vi "MotorControl_Test.vi"() -> ()   [LabVIEW 2020]
panel:
  out "Y Buffer":string
  in  "Y Axis Step Size":i32
  in  "Y Axis Range":i32
  out "Y Position":i32=2374 format="%b"
  out "Limit Switch Activated":bool
  out "Moving":bool
  out "Boolean Array":bool[](array[boolean])
  out "Binary Number":i32=2374 format="%b"
  in  "X Axis Step Size":i32
  in  "X Axis Range":i32
  in  "?":bool
  out "Angle Position":sgl
  out "X Position":sgl
  in  "Angle Step Size":i32
  in  "Angle Range":i32
  in  "?":refnum<k7>(container)
  out "X Translation Serial Number":i32=40849496
  in  "?":refnum<k7>(container)
  out "Angle Serial Number":i32=40808764
  # "Rotation Motor"
  # "Translation Motor"
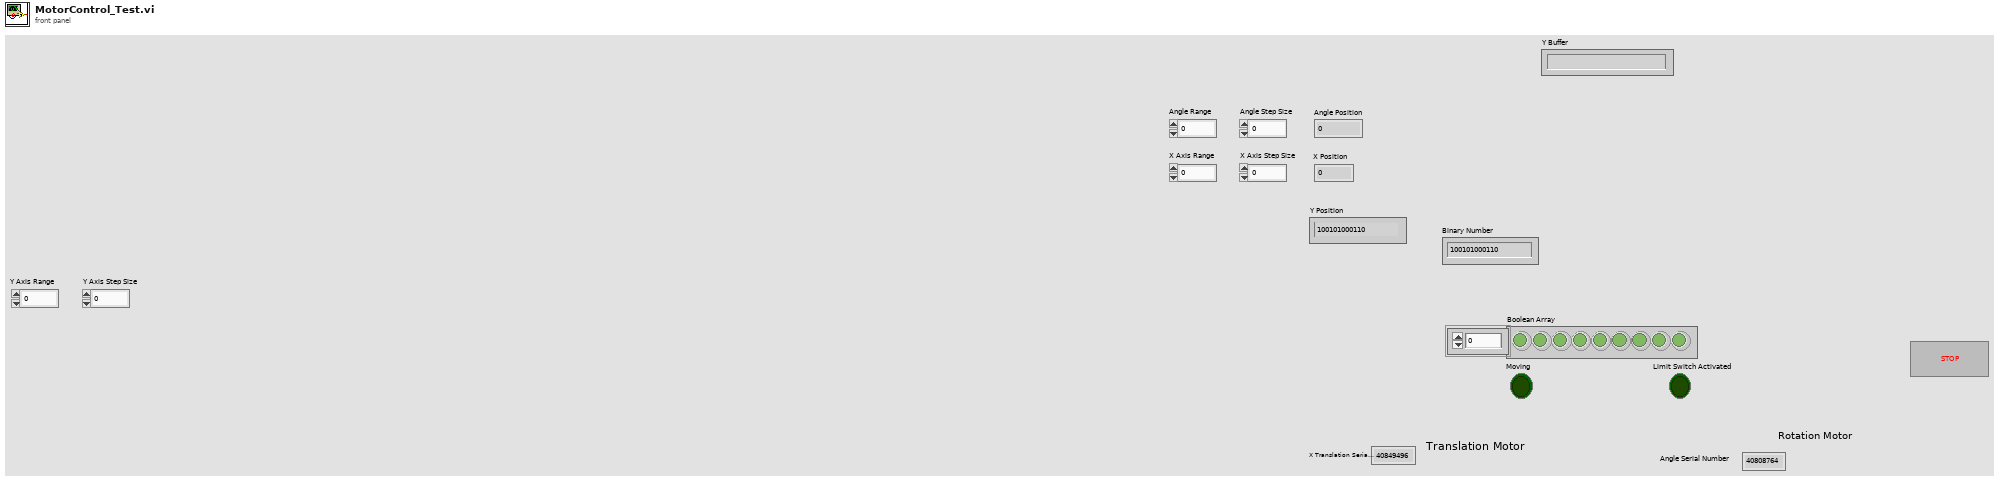
[diagram p1: front panel]
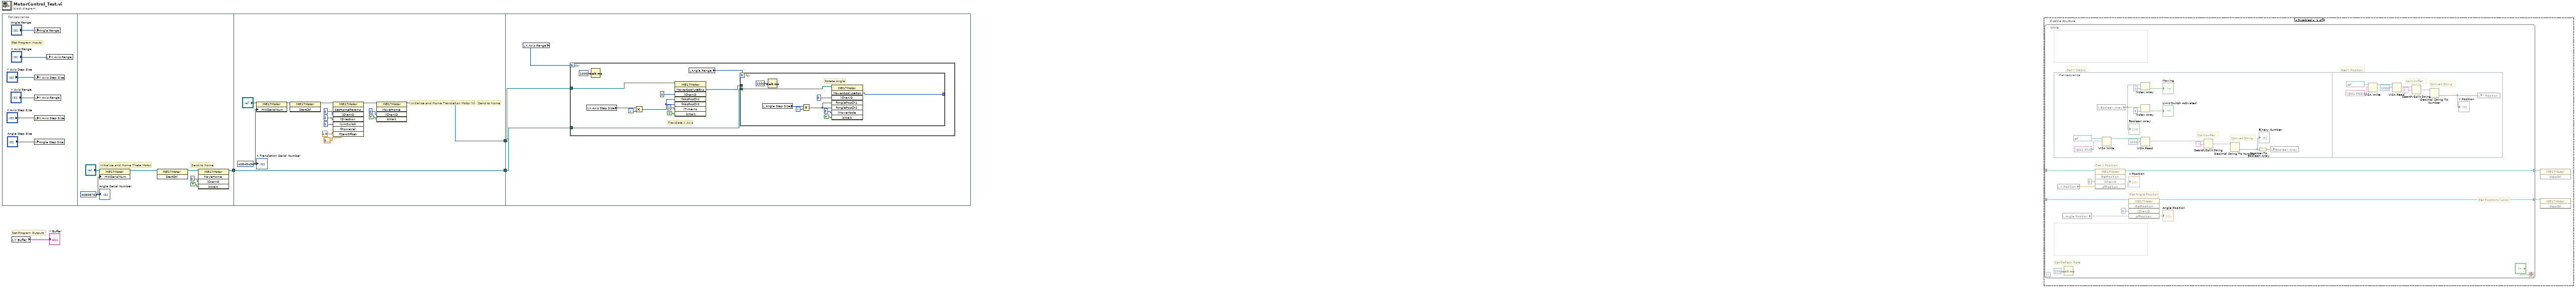
[diagram p0: block diagram]
diagram:
  # "Set Program Outputs"
  n1 = flat-sequence {
    tunnel: [w11] -> w4
    tunnel: w4 -> [w31]
    tunnel: [w31] -> w2
    tunnel: [w18] -> w1
    tunnel: w2 -> [w33]
    tunnel: w1 -> [w34]
    frame #0 {
      # "Get Program Inputs"
      n2 = local write "Angle Range"("Angle Range") -> ()
      n3 = local write "Y Axis Step Size"("Y Axis Step Size") -> ()
      n4 = local write "Y Axis Range"("Y Axis Range") -> ()
      n5 = local write "X Axis Step Size"("X Axis Step Size") -> ()
      n6 = local write "Angle Step Size"("Angle Step Size") -> ()
      n7 = local write "X Axis Range"("X Axis Range") -> ()
    }
    frame #1 {
      w12 = 40808764 ("Serial Number Number")
      # "Send to home"
      # "Initialise and Home Theta Motor"
      n8 = property on="Property Node" class="MG17Motor"(reference="?", "HWSerialNum"=w12) -> (reference out=w16:refnum<k7>)  [unwired: 1 in, 1 out]
      n9 = invoke class="MG17Motor" method="StartCtrl"(reference=w16) -> (reference out=w17:refnum<k7>)  [unwired: 2 in, 2 out]
      n10 = invoke class="MG17Motor" method="MoveHome"(reference=w17, "lChanID"=0, "bWait"=TRUE) -> (reference out=w11:refnum<k7>)  [unwired: 2 in, 4 out]
      "Angle Serial Number" <- w12
    }
    frame #2 {
      w19 = 40849496 ("Serial Number")
      # "Send to home"
      # "Initialise and Home Translation Motor (X)"
      n11 = property on="Property Node" class="MG17Motor"(reference="?", "HWSerialNum"=w19) -> (reference out=w27:refnum<k7>)  [unwired: 1 in, 1 out]
      n12 = invoke class="MG17Motor" method="StartCtrl"(reference=w27) -> (reference out=w29:refnum<k7>)  [unwired: 2 in, 2 out]
      n13 = invoke class="MG17Motor" method="SetHomeParams"(reference=w29, "lChanID"=0, "lDirection"=2, "lLimSwitch"=1, "fHomeVel"=sgl 1.0, "fZeroOffset"=sgl 0.1) -> (reference out=w30:refnum<k7>)  [unwired: 2 in, 7 out]
      n14 = invoke class="MG17Motor" method="MoveHome"(reference=w30, "lChanID"=0, "bWait"=TRUE) -> (reference out=w18:refnum<k7>)  [unwired: 2 in, 4 out]
      "X Translation Serial Number" <- w19
    }
    frame #3 {
      n15 = local read "X Axis Range"() -> (w32:i32)
      n16 = for {
        N: w32 -> [_]
        tunnel: w33 -> [w36]
        tunnel: w34 -> [w35]
        i -> [w40]
        # "Translate X Axis"
        n17 = local read "X Axis Step Size"() -> (w42:i32)
        n18 = Wait (ms)(milliseconds to wait=u32 1000) -> ()  [unwired: 1 out]
        n19 = Multiply(x=w42, y=w40) -> (x*y=w41:i32)
        n20 = invoke class="MG17Motor" method="MoveAbsoluteEnc"(reference=w35, "lChanID"=0, "fAbsPosCh1"=w41, "fAbsPosCh2"=w41, "lTimeInc"=1, "bWait"=TRUE) -> ("MoveAbsoluteEnc"=w37:i32)  [unwired: 2 in, 7 out]
        n21 = local read "Angle Range"() -> (w38:i32)
        n22 = for {
          N: w38 -> [_]
          tunnel: w37 -> [_]
          tunnel: [w46] -> _ mode=indexing
          tunnel: w36 -> [w47]
          i -> [w49]
          # "Rotate Angle"
          n23 = local read "Angle Step Size"() -> (w51:i32)
          n24 = Wait (ms)(milliseconds to wait=u32 1000) -> ()  [unwired: 1 out]
          n25 = Multiply(x=w51, y=w49) -> (x*y=w50:i32)
          n26 = invoke class="MG17Motor" method="MoveAbsoluteRot"(reference=w47, "lChanID"=0, "fAnglePosCh1"=w50, "fAnglePosCh2"=w50, "lMoveMode"=3 ("lTimeInc"), "bWait"=TRUE) -> ("MoveAbsoluteRot"=w46:i32)  [unwired: 2 in, 7 out]
        }
      }
    }
  }
  n27 = local read "Y Buffer"() -> (→"Y Buffer":string)
  n28 = disable-structure shown="Disabled" {
    frame Disabled {
      n29 = while {
        tunnel: [w67] -> w56
        tunnel: [w61] -> w55
        tunnel: _ -> [w58]
        tunnel: _ -> [w57]
        stop <- "?" stop-if-true
        # "Get Positions (Loop)"
        # "Get Y Position"
        # "Get Y Status"
        # "Get Angle Position"
        # "Get X Position"
        # "Set Refresh Rate"
        n30 = flat-sequence {
          frame #0 {
            # "Convert String"
            # "Split buffer"
            n31 = local read "Boolean Array"() -> (w70:bool[])
            "Boolean Array" <- w70
            n32 = VISA Write(VISA resource name=refnum<visa-resource-name> "COM3" ("VISA resource name out"), write buffer="@01 STAT" ("Command 2")) -> (VISA resource name out=w76:refnum<visa-resource-name>)  [unwired: 1 in, 2 out]
            n33 = Index Array(array=w70, index=0) -> (element=→"Moving":bool)
            n34 = Index Array(array=w70, index=8) -> (element=→"Limit Switch Activated":bool)
            n35 = VISA Read(VISA resource name=w76, byte count=u32 1000 ("Read Word Length Count?")) -> (read buffer=w77:string)  [unwired: 1 in, 3 out]
            n36 = Search/Split String(string=w77, search string/char (-)=" ") -> (match + rest of string=w80:string)  [unwired: 1 in, 2 out]
            n37 = Decimal String To Number(string=w80) -> (number=w78:i32)  [unwired: 2 in, 1 out]
            "Binary Number" <- w78
            n38 = Number To Boolean Array(number=w78) -> (Boolean array=w79:bool[])
            n39 = local write "Boolean Array"(w79) -> ()
          }
          frame #1 {
            # "Convert String"
            # "Split buffer"
            n40 = VISA Write(VISA resource name=refnum<visa-resource-name> "COM3" ("VISA resource name out"), write buffer="@01 POSN" ("Command 2")) -> (VISA resource name out=w90:refnum<visa-resource-name>)  [unwired: 1 in, 2 out]
            n41 = VISA Read(VISA resource name=w90, byte count=u32 1000 ("Read Word Length Count?")) -> (read buffer=w83:string)  [unwired: 1 in, 3 out]
            n42 = Search/Split String(string=w83, search string/char (-)=" ") -> (match + rest of string=w89:string)  [unwired: 1 in, 2 out]
            n43 = Decimal String To Number(string=w89) -> (number=w84:i32)  [unwired: 2 in, 1 out]
            "Y Position" <- w84
            n44 = local write "Y Position"(w84) -> ()
          }
        }
        n45 = local read "X Position"() -> (w59:sgl)
        n46 = local read "Angle Position"() -> (w60:sgl)
        n47 = Wait (ms)(milliseconds to wait=u32 200 ("millisecond timer value")) -> ()  [unwired: 1 out]
        n48 = invoke class="MG17Motor" method="GetPosition"(reference=w58, "lChanID"=0, "pfPosition"=w59) -> (reference out=w61:refnum<k7>, "pfPosition"=→"X Position":sgl)  [unwired: 2 in, 3 out]
        n49 = invoke class="MG17Motor" method="GetPosition"(reference=w57, "lChanID"=0, "pfPosition"=w60) -> (reference out=w67:refnum<k7>, "pfPosition"=→"Angle Position":sgl)  [unwired: 2 in, 3 out]
      }
      n50 = invoke class="MG17Motor" method="StopCtrl"(reference=w55) -> ()  [unwired: 2 in, 3 out]
      n51 = invoke class="MG17Motor" method="StopCtrl"(reference=w56) -> ()  [unwired: 2 in, 3 out]
    }
    frame Enabled {
    }
  }
